vi "DIselector.vi"(8 "I/O element":T1(ring)) -> (3 "value":bool)   [LabVIEW 2014]
uses:
  <vilib>/rvi/eio/common/nirviEmuTemplateMethod_errors.vi
  <vilib>/eio/EIONode/EIONode.xnode
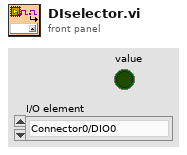
[diagram p1: front panel]
types:
  T1 = enum16{"Connector0/DIO0", "Connector0/DIO1", "Connector0/DIO2", "Connector0/DIO3", "Connector0/DIO4", "Connector0/DIO5", "Connector0/DIO6", "Connector0/DIO7", "Connector0/DIO8", "Connector0/DIO9", "Connector0/DIO10", "Connector0/DIO11", "Connector0/DIO12", "Connector0/DIO13", "Connector0/DIO14", "Connector0/DIO15", "Connector1/DIO0", "Connector1/DIO1", "Connector1/DIO2", "Connector1/DIO3", "Connector1/DIO4", "Connector1/DIO5", "Connector1/DIO6", "Connector1/DIO7", "Connector1/DIO8", "Connector1/DIO9", "Connector1/DIO10", "Connector1/DIO11", "Connector1/DIO12", "Connector1/DIO13", "Connector1/DIO14", "Connector1/DIO15", "Connector1/DIO16", "Connector1/DIO17", "Connector1/DIO18", "Connector1/DIO19", "Connector1/DIO20", "Connector1/DIO21", "Connector1/DIO22", "Connector1/DIO23", "Connector1/DIO24", "Connector1/DIO25", "Connector1/DIO26", "Connector1/DIO27", "Connector1/DIO28", "Connector1/DIO29", "Connector1/DIO30", "Connector1/DIO31", "Connector1/DIO32", "Connector1/DIO33", "Connector1/DIO34", "Connector1/DIO35", "Connector1/DIO36", "Connector1/DIO37", "Connector1/DIO38", "Connector1/DIO39", "Connector2/DIO0", "Connector2/DIO1", "Connector2/DIO2", "Connector2/DIO3", "Connector2/DIO4", "Connector2/DIO5", "Connector2/DIO6", "Connector2/DIO7", "Connector2/DIO8", "Connector2/DIO9", "Connector2/DIO10", "Connector2/DIO11", "Connector2/DIO12", "Connector2/DIO13", "Connector2/DIO14", "Connector2/DIO15", "Connector2/DIO16", "Connector2/DIO17", "Connector2/DIO18", "Connector2/DIO19", "Connector2/DIO20", "Connector2/DIO21", "Connector2/DIO22", "Connector2/DIO23", "Connector2/DIO24", "Connector2/DIO25", "Connector2/DIO26", "Connector2/DIO27", "Connector2/DIO28", "Connector2/DIO29", "Connector2/DIO30", "Connector2/DIO31", "Connector2/DIO32", "Connector2/DIO33", "Connector2/DIO34", "Connector2/DIO35", "Connector2/DIO36", "Connector2/DIO37", "Connector2/DIO38", "Connector2/DIO39"}
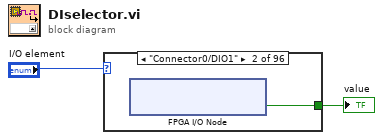
[diagram p0: block diagram]
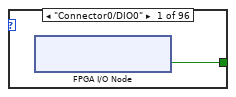
[diagram p2: hidden frame]
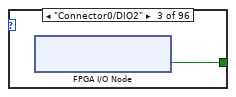
[diagram p3: hidden frame]
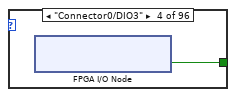
[diagram p4: hidden frame]
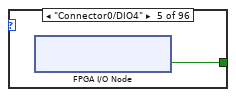
[diagram p5: hidden frame]
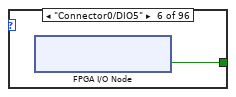
[diagram p6: hidden frame]
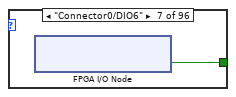
[diagram p7: hidden frame]
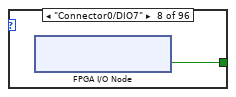
[diagram p8: hidden frame]
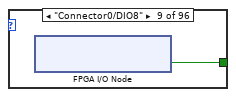
[diagram p9: hidden frame]
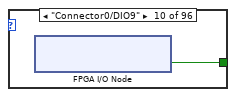
[diagram p10: hidden frame]
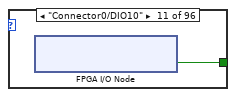
[diagram p11: hidden frame]
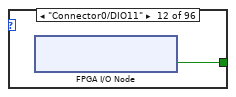
[diagram p12: hidden frame]
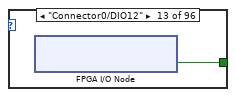
[diagram p13: hidden frame]
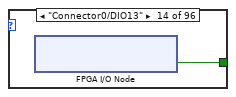
[diagram p14: hidden frame]
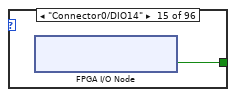
[diagram p15: hidden frame]
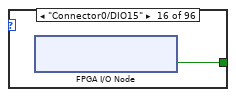
[diagram p16: hidden frame]
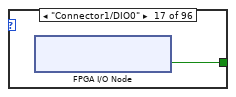
[diagram p17: hidden frame]
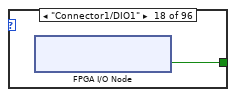
[diagram p18: hidden frame]
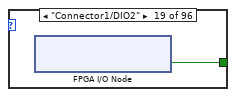
[diagram p19: hidden frame]
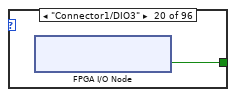
[diagram p20: hidden frame]
diagram:
  n1 = case shown="\"Connector0/DIO1\"" "I/O element" {
    tunnel: [w3 w4 w5 w6 w7 w8 w9 w10 w11 w12 w13 w14 w15 w16 w17 w18 w19 w20 w21 w22 w23 w24 w25 w26 w27 w28 w29 w30 w31 w32 w33 w34 w35 w36 w37 w38 w39 w40 w41 w42 w43 w44 w45 w46 w47 w48 w49 w50 w51 w52 w53 w54 w55 w56 w57 w58 w59 w60 w61 w62 w63 w64 w65 w66 w67 w68 w69 w70 w71 w72 w73 w74 w75 w76 w77 w78 w79 w80 w81 w82 w83 w84 w85 w86 w87 w88 w89 w90 w91 w92 w93 w94 w95 w96 w97 w98] -> w1
    frame "Connector0/DIO0" {
      n2 = xnode "FPGA I/O Node"() -> ("Connector0/DIO0"=w3:bool)  [unwired: 1 in, 1 out]
    }
    frame "Connector0/DIO1" {
      n3 = xnode "FPGA I/O Node"() -> ("Connector0/DIO1"=w4:bool)  [unwired: 1 in, 1 out]
    }
    frame "Connector0/DIO2" {
      n4 = xnode "FPGA I/O Node"() -> ("Connector0/DIO2"=w5:bool)  [unwired: 1 in, 1 out]
    }
    frame "Connector0/DIO3" {
      n5 = xnode "FPGA I/O Node"() -> ("Connector0/DIO3"=w6:bool)  [unwired: 1 in, 1 out]
    }
    frame "Connector0/DIO4" {
      n6 = xnode "FPGA I/O Node"() -> ("Connector0/DIO4"=w7:bool)  [unwired: 1 in, 1 out]
    }
    frame "Connector0/DIO5" {
      n7 = xnode "FPGA I/O Node"() -> ("Connector0/DIO5"=w8:bool)  [unwired: 1 in, 1 out]
    }
    frame "Connector0/DIO6" {
      n8 = xnode "FPGA I/O Node"() -> ("Connector0/DIO6"=w9:bool)  [unwired: 1 in, 1 out]
    }
    frame "Connector0/DIO7" {
      n9 = xnode "FPGA I/O Node"() -> ("Connector0/DIO7"=w10:bool)  [unwired: 1 in, 1 out]
    }
    frame "Connector0/DIO8" {
      n10 = xnode "FPGA I/O Node"() -> ("Connector0/DIO8"=w11:bool)  [unwired: 1 in, 1 out]
    }
    frame "Connector0/DIO9" {
      n11 = xnode "FPGA I/O Node"() -> ("Connector0/DIO9"=w12:bool)  [unwired: 1 in, 1 out]
    }
    frame "Connector0/DIO10" {
      n12 = xnode "FPGA I/O Node"() -> ("Connector0/DIO10"=w13:bool)  [unwired: 1 in, 1 out]
    }
    frame "Connector0/DIO11" {
      n13 = xnode "FPGA I/O Node"() -> ("Connector0/DIO11"=w14:bool)  [unwired: 1 in, 1 out]
    }
    frame "Connector0/DIO12" {
      n14 = xnode "FPGA I/O Node"() -> ("Connector0/DIO12"=w15:bool)  [unwired: 1 in, 1 out]
    }
    frame "Connector0/DIO13" {
      n15 = xnode "FPGA I/O Node"() -> ("Connector0/DIO13"=w16:bool)  [unwired: 1 in, 1 out]
    }
    frame "Connector0/DIO14" {
      n16 = xnode "FPGA I/O Node"() -> ("Connector0/DIO14"=w17:bool)  [unwired: 1 in, 1 out]
    }
    frame "Connector0/DIO15" {
      n17 = xnode "FPGA I/O Node"() -> ("Connector0/DIO15"=w18:bool)  [unwired: 1 in, 1 out]
    }
    frame "Connector1/DIO0" {
      n18 = xnode "FPGA I/O Node"() -> ("Connector1/DIO0"=w19:bool)  [unwired: 1 in, 1 out]
    }
    frame "Connector1/DIO1" {
      n19 = xnode "FPGA I/O Node"() -> ("Connector1/DIO1"=w20:bool)  [unwired: 1 in, 1 out]
    }
    frame "Connector1/DIO2" {
      n20 = xnode "FPGA I/O Node"() -> ("Connector1/DIO2"=w21:bool)  [unwired: 1 in, 1 out]
    }
    frame "Connector1/DIO3" {
      n21 = xnode "FPGA I/O Node"() -> ("Connector1/DIO3"=w22:bool)  [unwired: 1 in, 1 out]
    }
    frame "Connector1/DIO4" {
      n22 = xnode "FPGA I/O Node"() -> ("Connector1/DIO4"=w23:bool)  [unwired: 1 in, 1 out]
    }
    frame "Connector1/DIO5" {
      n23 = xnode "FPGA I/O Node"() -> ("Connector1/DIO5"=w24:bool)  [unwired: 1 in, 1 out]
    }
    frame "Connector1/DIO6" {
      n24 = xnode "FPGA I/O Node"() -> ("Connector1/DIO6"=w25:bool)  [unwired: 1 in, 1 out]
    }
    frame "Connector1/DIO7" {
      n25 = xnode "FPGA I/O Node"() -> ("Connector1/DIO7"=w26:bool)  [unwired: 1 in, 1 out]
    }
    frame "Connector1/DIO8" {
      n26 = xnode "FPGA I/O Node"() -> ("Connector1/DIO8"=w27:bool)  [unwired: 1 in, 1 out]
    }
    frame "Connector1/DIO9" {
      n27 = xnode "FPGA I/O Node"() -> ("Connector1/DIO9"=w28:bool)  [unwired: 1 in, 1 out]
    }
    frame "Connector1/DIO10" {
      n28 = xnode "FPGA I/O Node"() -> ("Connector1/DIO10"=w29:bool)  [unwired: 1 in, 1 out]
    }
    frame "Connector1/DIO11" {
      n29 = xnode "FPGA I/O Node"() -> ("Connector1/DIO11"=w30:bool)  [unwired: 1 in, 1 out]
    }
    frame "Connector1/DIO12" {
      n30 = xnode "FPGA I/O Node"() -> ("Connector1/DIO12"=w31:bool)  [unwired: 1 in, 1 out]
    }
    frame "Connector1/DIO13" {
      n31 = xnode "FPGA I/O Node"() -> ("Connector1/DIO13"=w32:bool)  [unwired: 1 in, 1 out]
    }
    frame "Connector1/DIO14" {
      n32 = xnode "FPGA I/O Node"() -> ("Connector1/DIO14"=w33:bool)  [unwired: 1 in, 1 out]
    }
    frame "Connector1/DIO15" {
      n33 = xnode "FPGA I/O Node"() -> ("Connector1/DIO15"=w34:bool)  [unwired: 1 in, 1 out]
    }
    frame "Connector1/DIO16" {
      n34 = xnode "FPGA I/O Node"() -> ("Connector1/DIO16"=w35:bool)  [unwired: 1 in, 1 out]
    }
    frame "Connector1/DIO17" {
      n35 = xnode "FPGA I/O Node"() -> ("Connector1/DIO17"=w36:bool)  [unwired: 1 in, 1 out]
    }
    frame "Connector1/DIO18" {
      n36 = xnode "FPGA I/O Node"() -> ("Connector1/DIO18"=w37:bool)  [unwired: 1 in, 1 out]
    }
    frame "Connector1/DIO19" {
      n37 = xnode "FPGA I/O Node"() -> ("Connector1/DIO19"=w38:bool)  [unwired: 1 in, 1 out]
    }
    frame "Connector1/DIO20" {
      n38 = xnode "FPGA I/O Node"() -> ("Connector1/DIO20"=w39:bool)  [unwired: 1 in, 1 out]
    }
    frame "Connector1/DIO21" {
      n39 = xnode "FPGA I/O Node"() -> ("Connector1/DIO21"=w40:bool)  [unwired: 1 in, 1 out]
    }
    frame "Connector1/DIO22" {
      n40 = xnode "FPGA I/O Node"() -> ("Connector1/DIO22"=w41:bool)  [unwired: 1 in, 1 out]
    }
    frame "Connector1/DIO23" {
      n41 = xnode "FPGA I/O Node"() -> ("Connector1/DIO23"=w42:bool)  [unwired: 1 in, 1 out]
    }
    frame "Connector1/DIO24" {
      n42 = xnode "FPGA I/O Node"() -> ("Connector1/DIO24"=w43:bool)  [unwired: 1 in, 1 out]
    }
    frame "Connector1/DIO25" {
      n43 = xnode "FPGA I/O Node"() -> ("Connector1/DIO25"=w44:bool)  [unwired: 1 in, 1 out]
    }
    frame "Connector1/DIO26" {
      n44 = xnode "FPGA I/O Node"() -> ("Connector1/DIO26"=w45:bool)  [unwired: 1 in, 1 out]
    }
    frame "Connector1/DIO27" {
      n45 = xnode "FPGA I/O Node"() -> ("Connector1/DIO27"=w46:bool)  [unwired: 1 in, 1 out]
    }
    frame "Connector1/DIO28" {
      n46 = xnode "FPGA I/O Node"() -> ("Connector1/DIO28"=w47:bool)  [unwired: 1 in, 1 out]
    }
    frame "Connector1/DIO29" {
      n47 = xnode "FPGA I/O Node"() -> ("Connector1/DIO29"=w48:bool)  [unwired: 1 in, 1 out]
    }
    frame "Connector1/DIO30" {
      n48 = xnode "FPGA I/O Node"() -> ("Connector1/DIO30"=w49:bool)  [unwired: 1 in, 1 out]
    }
    frame "Connector1/DIO31" {
      n49 = xnode "FPGA I/O Node"() -> ("Connector1/DIO31"=w50:bool)  [unwired: 1 in, 1 out]
    }
    frame "Connector1/DIO32" {
      n50 = xnode "FPGA I/O Node"() -> ("Connector1/DIO32"=w51:bool)  [unwired: 1 in, 1 out]
    }
    frame "Connector1/DIO33" {
      n51 = xnode "FPGA I/O Node"() -> ("Connector1/DIO33"=w52:bool)  [unwired: 1 in, 1 out]
    }
    frame "Connector1/DIO34" {
      n52 = xnode "FPGA I/O Node"() -> ("Connector1/DIO34"=w53:bool)  [unwired: 1 in, 1 out]
    }
    frame "Connector1/DIO35" {
      n53 = xnode "FPGA I/O Node"() -> ("Connector1/DIO35"=w54:bool)  [unwired: 1 in, 1 out]
    }
    frame "Connector1/DIO36" {
      n54 = xnode "FPGA I/O Node"() -> ("Connector1/DIO36"=w55:bool)  [unwired: 1 in, 1 out]
    }
    frame "Connector1/DIO37" {
      n55 = xnode "FPGA I/O Node"() -> ("Connector1/DIO37"=w56:bool)  [unwired: 1 in, 1 out]
    }
    frame "Connector1/DIO38" {
      n56 = xnode "FPGA I/O Node"() -> ("Connector1/DIO38"=w57:bool)  [unwired: 1 in, 1 out]
    }
    frame "Connector1/DIO39" {
      n57 = xnode "FPGA I/O Node"() -> ("Connector1/DIO39"=w58:bool)  [unwired: 1 in, 1 out]
    }
    frame "Connector2/DIO0" {
      n58 = xnode "FPGA I/O Node"() -> ("Connector2/DIO0"=w59:bool)  [unwired: 1 in, 1 out]
    }
    frame "Connector2/DIO1" {
      n59 = xnode "FPGA I/O Node"() -> ("Connector2/DIO1"=w60:bool)  [unwired: 1 in, 1 out]
    }
    frame "Connector2/DIO2" {
      n60 = xnode "FPGA I/O Node"() -> ("Connector2/DIO2"=w61:bool)  [unwired: 1 in, 1 out]
    }
    frame "Connector2/DIO3" {
      n61 = xnode "FPGA I/O Node"() -> ("Connector2/DIO3"=w62:bool)  [unwired: 1 in, 1 out]
    }
    frame "Connector2/DIO4" {
      n62 = xnode "FPGA I/O Node"() -> ("Connector2/DIO4"=w63:bool)  [unwired: 1 in, 1 out]
    }
    frame "Connector2/DIO5" {
      n63 = xnode "FPGA I/O Node"() -> ("Connector2/DIO5"=w64:bool)  [unwired: 1 in, 1 out]
    }
    frame "Connector2/DIO6" {
      n64 = xnode "FPGA I/O Node"() -> ("Connector2/DIO6"=w65:bool)  [unwired: 1 in, 1 out]
    }
    frame "Connector2/DIO7" {
      n65 = xnode "FPGA I/O Node"() -> ("Connector2/DIO7"=w66:bool)  [unwired: 1 in, 1 out]
    }
    frame "Connector2/DIO8" {
      n66 = xnode "FPGA I/O Node"() -> ("Connector2/DIO8"=w67:bool)  [unwired: 1 in, 1 out]
    }
    frame "Connector2/DIO9" {
      n67 = xnode "FPGA I/O Node"() -> ("Connector2/DIO9"=w68:bool)  [unwired: 1 in, 1 out]
    }
    frame "Connector2/DIO10" {
      n68 = xnode "FPGA I/O Node"() -> ("Connector2/DIO10"=w69:bool)  [unwired: 1 in, 1 out]
    }
    frame "Connector2/DIO11" {
      n69 = xnode "FPGA I/O Node"() -> ("Connector2/DIO11"=w70:bool)  [unwired: 1 in, 1 out]
    }
    frame "Connector2/DIO12" {
      n70 = xnode "FPGA I/O Node"() -> ("Connector2/DIO12"=w71:bool)  [unwired: 1 in, 1 out]
    }
    frame "Connector2/DIO13" {
      n71 = xnode "FPGA I/O Node"() -> ("Connector2/DIO13"=w72:bool)  [unwired: 1 in, 1 out]
    }
    frame "Connector2/DIO14" {
      n72 = xnode "FPGA I/O Node"() -> ("Connector2/DIO14"=w73:bool)  [unwired: 1 in, 1 out]
    }
    frame "Connector2/DIO15" {
      n73 = xnode "FPGA I/O Node"() -> ("Connector2/DIO15"=w74:bool)  [unwired: 1 in, 1 out]
    }
    frame "Connector2/DIO16" {
      n74 = xnode "FPGA I/O Node"() -> ("Connector2/DIO16"=w75:bool)  [unwired: 1 in, 1 out]
    }
    frame "Connector2/DIO17" {
      n75 = xnode "FPGA I/O Node"() -> ("Connector2/DIO17"=w76:bool)  [unwired: 1 in, 1 out]
    }
    frame "Connector2/DIO18" {
      n76 = xnode "FPGA I/O Node"() -> ("Connector2/DIO18"=w77:bool)  [unwired: 1 in, 1 out]
    }
    frame "Connector2/DIO19" {
      n77 = xnode "FPGA I/O Node"() -> ("Connector2/DIO19"=w78:bool)  [unwired: 1 in, 1 out]
    }
    frame "Connector2/DIO20" {
      n78 = xnode "FPGA I/O Node"() -> ("Connector2/DIO20"=w79:bool)  [unwired: 1 in, 1 out]
    }
    frame "Connector2/DIO21" {
      n79 = xnode "FPGA I/O Node"() -> ("Connector2/DIO21"=w80:bool)  [unwired: 1 in, 1 out]
    }
    frame "Connector2/DIO22" {
      n80 = xnode "FPGA I/O Node"() -> ("Connector2/DIO22"=w81:bool)  [unwired: 1 in, 1 out]
    }
    frame "Connector2/DIO23" {
      n81 = xnode "FPGA I/O Node"() -> ("Connector2/DIO23"=w82:bool)  [unwired: 1 in, 1 out]
    }
    frame "Connector2/DIO24" {
      n82 = xnode "FPGA I/O Node"() -> ("Connector2/DIO24"=w83:bool)  [unwired: 1 in, 1 out]
    }
    frame "Connector2/DIO25" {
      n83 = xnode "FPGA I/O Node"() -> ("Connector2/DIO25"=w84:bool)  [unwired: 1 in, 1 out]
    }
    frame "Connector2/DIO26" {
      n84 = xnode "FPGA I/O Node"() -> ("Connector2/DIO26"=w85:bool)  [unwired: 1 in, 1 out]
    }
    frame "Connector2/DIO27" {
      n85 = xnode "FPGA I/O Node"() -> ("Connector2/DIO27"=w86:bool)  [unwired: 1 in, 1 out]
    }
    frame "Connector2/DIO28" {
      n86 = xnode "FPGA I/O Node"() -> ("Connector2/DIO28"=w87:bool)  [unwired: 1 in, 1 out]
    }
    frame "Connector2/DIO29" {
      n87 = xnode "FPGA I/O Node"() -> ("Connector2/DIO29"=w88:bool)  [unwired: 1 in, 1 out]
    }
    frame "Connector2/DIO30" {
      n88 = xnode "FPGA I/O Node"() -> ("Connector2/DIO30"=w89:bool)  [unwired: 1 in, 1 out]
    }
    frame "Connector2/DIO31" {
      n89 = xnode "FPGA I/O Node"() -> ("Connector2/DIO31"=w90:bool)  [unwired: 1 in, 1 out]
    }
    frame "Connector2/DIO32" {
      n90 = xnode "FPGA I/O Node"() -> ("Connector2/DIO32"=w91:bool)  [unwired: 1 in, 1 out]
    }
    frame "Connector2/DIO33" {
      n91 = xnode "FPGA I/O Node"() -> ("Connector2/DIO33"=w92:bool)  [unwired: 1 in, 1 out]
    }
    frame "Connector2/DIO34" {
      n92 = xnode "FPGA I/O Node"() -> ("Connector2/DIO34"=w93:bool)  [unwired: 1 in, 1 out]
    }
    frame "Connector2/DIO35" {
      n93 = xnode "FPGA I/O Node"() -> ("Connector2/DIO35"=w94:bool)  [unwired: 1 in, 1 out]
    }
    frame "Connector2/DIO36" {
      n94 = xnode "FPGA I/O Node"() -> ("Connector2/DIO36"=w95:bool)  [unwired: 1 in, 1 out]
    }
    frame "Connector2/DIO37" {
      n95 = xnode "FPGA I/O Node"() -> ("Connector2/DIO37"=w96:bool)  [unwired: 1 in, 1 out]
    }
    frame "Connector2/DIO38" {
      n96 = xnode "FPGA I/O Node"() -> ("Connector2/DIO38"=w97:bool)  [unwired: 1 in, 1 out]
    }
    frame "Connector2/DIO39" {
      n97 = xnode "FPGA I/O Node"() -> ("Connector2/DIO39"=w98:bool)  [unwired: 1 in, 1 out]
    }
  }
  "value" <- w1
